vi "read Double.vi"(10 "index":i32, 11 "data table in":T1) -> (1 "value":dbl, 3 "data table out":T1)   [LabVIEW 2013, in "data bus values.lvlib"]
doc: "Reads a single value from the data table."
uses:
  data bus values.lvlib
  data table.ctl
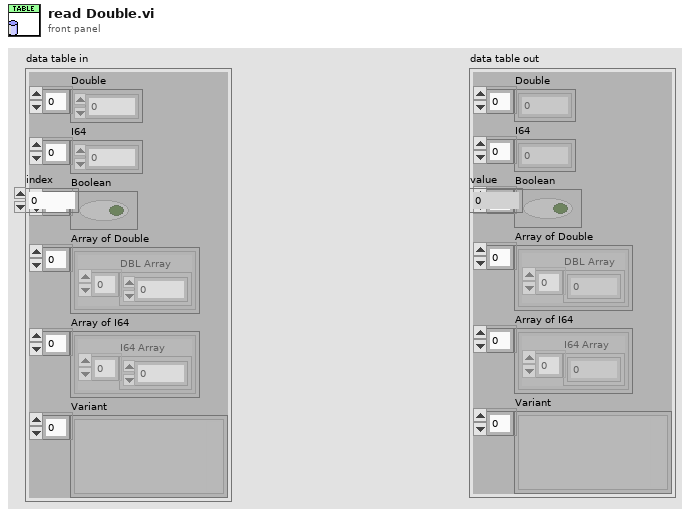
[diagram p1: front panel]
types:
  T1 = typedef "data bus values.lvlib/data table.ctl" = cluster{"Double":dbl[], "I64":i64[], "Boolean":bool[], "Array of Double":cluster{"DBL Array":dbl[]}[], "Array of I64":cluster{"I64 Array":i64[]}[], "Variant":variant[]}
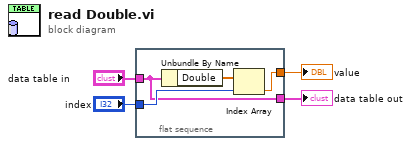
[diagram p0: block diagram]
diagram:
  n1 = flat-sequence {
    tunnel: "index" -> [w8]
    tunnel: [w7] -> w3
    tunnel: "data table in" -> [w5]
    tunnel: [w5] -> w1
    frame #0 {
      n2 = Unbundle By Name(w5) -> ("Double"=w6:dbl[])
      n3 = Index Array(array=w6, index=w8) -> (element=w7:dbl)
    }
  }
  "data table out" <- w1
  "value" <- w3
